vi "Display Info.vi"(7 "Layout ref":refnum<vi>, 8 "error in (no error)":errorcluster, 9 "Modify (F) /Add [T]":bool, 10 "Names in use":string[](array[string]), 11 "ArduinoDAC in":refnum<class "ArduinoDAC.lvclass">) -> (0 "error out":errorcluster, 1 "Names in use out":string[](array[string]), 2 "Changes Made?":bool, 3 "ArduinoDAC out":refnum<class "ArduinoDAC.lvclass">)   [LabVIEW 2013, in "ArduinoDAC.lvclass"]
uses:
  ArduinoDAC.lvclass
  TypeDefs/ColumnAppearCluster.ctl
  ArduinoDAC.lvclass/ArduinoDAC.ctl
  ColumnVIs/Column/Column.lvclass
panel:
  in  "Steps Column Appearance":T1={"Column Name"="Frequency", "Width"=30, "Bkgd"=[16448250], "Text"=[0]}
  in  "EndV Column Appearance":T1={"Column Name"="Frequency", "Width"=30, "Bkgd"=[16448250], "Text"=[0]}
  in  "StartV Column Appearance":T1={"Column Name"="Frequency", "Width"=30, "Bkgd"=[16448250], "Text"=[0]}
  in  "Device Description":string
  in  "Hardware Settings":T2={"PB Trigger Line"=65535, "Serial Port"=""}
  in  "Name":string
  in  "Done":bool
  in  "Cancel":bool
  # "This VI just sets the wiring structure.\nOpen a child override version instead!"
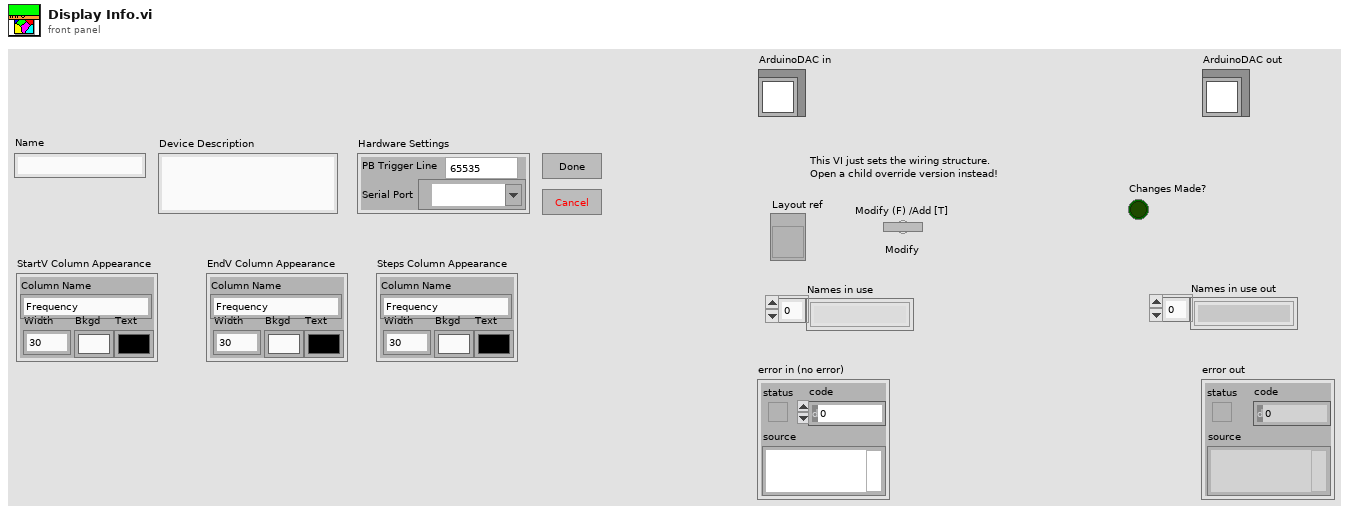
[diagram p1: front panel]
types:
  T1 = typedef "ColumnAppearCluster.ctl" = cluster{"Column Name":string, "Width":u32, "Bkgd":u32[], "Text":u32[]}
  T2 = cluster{"PB Trigger Line":u16, "Serial Port":refnum<visa-resource-name>}
  T3 = cluster{u16, "Serial Port":refnum<visa-resource-name>}
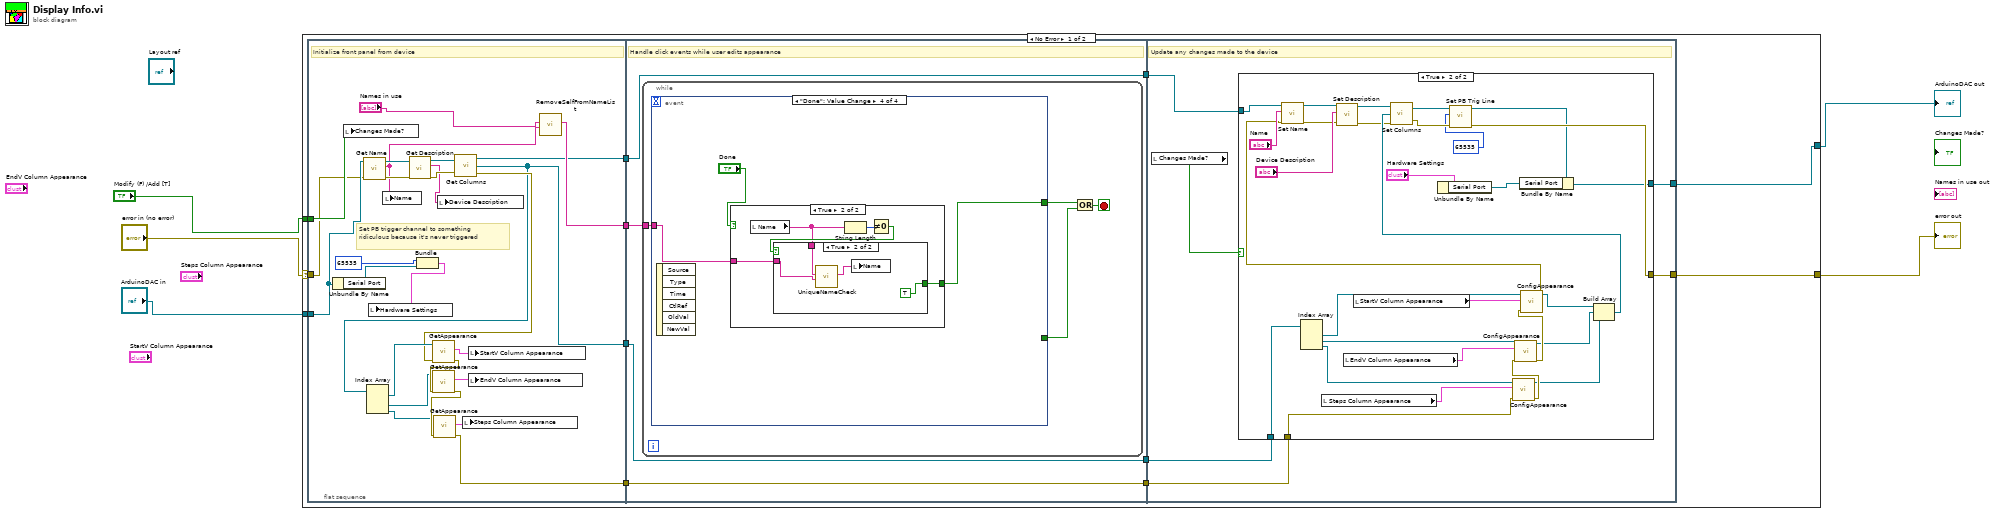
[diagram p0: block diagram]
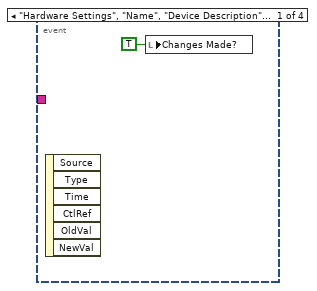
[diagram p2: hidden frame]
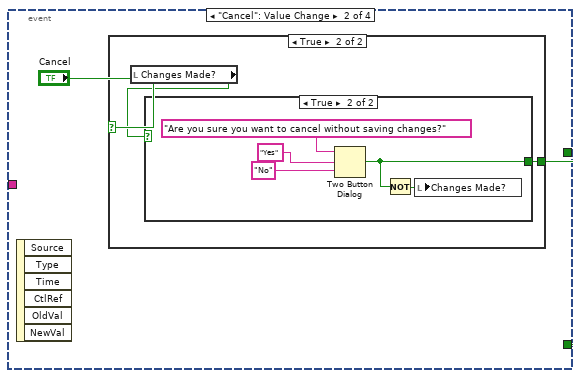
[diagram p3: hidden frame]
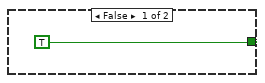
[diagram p5: hidden frame]
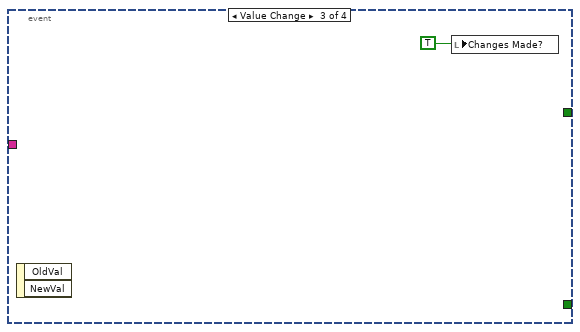
[diagram p6: hidden frame]
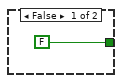
[diagram p7: hidden frame]
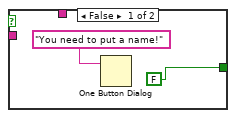
[diagram p8: hidden frame]
diagram:
  n1 = case shown="No Error" "error in (no error)" {
    selector: "error in (no error)" -> [w15 w119]
    tunnel: [w7 w119] -> w1
    tunnel: [w6 w118] -> w2
    tunnel: "ArduinoDAC in" -> [w16 w118]
    tunnel: "Modify (F) /Add [T]" -> [w17 _]
    frame No Error {
      n2 = flat-sequence {
        tunnel: w17 -> [w43]
        tunnel: w16 -> [w39]
        tunnel: w15 -> [w37]
        tunnel: [w28] -> w14
        tunnel: [w27] -> w13
        tunnel: [w26] -> w11
        tunnel: [w20] -> w9
        tunnel: w14 -> [w47]
        tunnel: w13 -> [w46]
        tunnel: [w46] -> w12
        tunnel: w11 -> [w45]
        tunnel: [w45] -> w10
        tunnel: w9 -> [w44]
        tunnel: [w44] -> w8
        tunnel: w12 -> [w85]
        tunnel: w10 -> [w84]
        tunnel: w8 -> [w83]
        tunnel: [w81] -> w7
        tunnel: [w80] -> w6
        frame #0 {
          # "Set PB trigger channel to something ridiculous because it's never triggered"
          # "Initialize front panel from device"
          n3 = Unbundle By Name(w39) -> ("Serial Port"=w41:refnum<visa-resource-name>)
          n4 = local write "Changes Made?"(w43) -> ()
          n5 = call-dynamic "Get Name.vi"("error in (no error)"=w37, "Device in"=w39) -> ("error out"=w36:errorcluster, "Name"=w33:string, "Device out"=w38:refnum<class "ArduinoDAC.lvclass">)  [unwired: 7 in]
          n6 = local write "Name"(w33) -> ()
          n7 = call-dynamic "Get Description.vi"("error in (no error)"=w36, "Device in"=w38) -> ("error out"=w34:errorcluster, "Device Description"=w32:string, "Device out"=w35:refnum<class "ArduinoDAC.lvclass">)  [unwired: 7 in]
          n8 = Bundle(u16 65535, "Serial Port"=w41) -> (w40:T3)  [unwired: 1 in]
          n9 = local write "Hardware Settings"(w40) -> ()
          n10 = local write "Device Description"(w32) -> ()
          n11 = call-dynamic "Get Columns.vi"("Device in"=w35, "error in (no error)"=w34) -> ("Device out"=w27:refnum<class "ArduinoDAC.lvclass">, "Columns"=w26:refnum<class "Column.lvclass">[], "error out"=w30:errorcluster)
          n12 = Index Array(array=w26) -> (element #1=w31:refnum<class "Column.lvclass">, element #2=w23:refnum<class "Column.lvclass">, element #3=w21:refnum<class "Column.lvclass">)  [unwired: 3 in]
          n13 = call "GetAppearance.vi"("error in (no error)"=w30, "Column in"=w31) -> ("error out"=w24:errorcluster, "Column Appearance"=w29:T1)  [unwired: 7 in, 1 out]
          n14 = call "GetAppearance.vi"("error in (no error)"=w24, "Column in"=w23) -> ("error out"=w22:errorcluster, "Column Appearance"=w19:T1)  [unwired: 7 in, 1 out]
          n15 = call "GetAppearance.vi"("error in (no error)"=w22, "Column in"=w21) -> ("error out"=w20:errorcluster, "Column Appearance"=w18:T1)  [unwired: 7 in, 1 out]
          n16 = local write "Steps Column Appearance"(w18) -> ()
          n17 = local write "StartV Column Appearance"(w29) -> ()
          n18 = local write "EndV Column Appearance"(w19) -> ()
          n19 = call "RemoveSelfFromNameList.vi"("self Name"=w33, "Names in use"="Names in use") -> ("Reserved Names"=w28:string[])  [unwired: 9 in]
        }
        frame #1 {
          # "Handle click events while user edits appearance"
          n20 = while {
            tunnel: w47 -> [w48]
            stop <- w51 stop-if-true
            n21 = event shown="[3] \"Done\": Value Change" {
              selector: _ -> [_ _ _ _]
              dyn-events: _ -> [_ _ _ _]
              timeout: _ -> [_ _ _ _]
              tunnel: [_ w54 _ _] -> w50
              tunnel: [_ _ _ w67] -> w49
              tunnel: w48 -> [_ _ _ w65]
              event "Hardware Settings", "Name", "Device Description": Value Change {
                n22 = event-data() -> ()  [unwired: 1 in, 6 out]
                n23 = local write "Changes Made?"(TRUE ("Changes Made?")) -> ()
              }
              event "Cancel": Value Change {
                n24 = event-data() -> ()  [unwired: 1 in, 6 out]
                n25 = case shown="True" "Cancel" {
                  selector: "Cancel" -> [w55 _]
                  tunnel: [w55 w57] -> w54
                  frame False {
                  }
                  frame True {
                    n26 = local read "Changes Made?"() -> (w56:bool)
                    n27 = case shown="True" w56 {
                      tunnel: [TRUE w60] -> w57
                      frame False {
                      }
                      frame True {
                        n28 = Two Button Dialog(message="Are you sure you want to cancel without saving changes?", 1:"No", 2:"Yes") -> (T button?=w60:bool)
                        n29 = Not(x=w60) -> (.not. x?=w59:bool)
                        n30 = local write "Changes Made?"(w59) -> ()
                      }
                    }
                  }
                }
              }
              event Value Change {
                n31 = event-data() -> ()  [unwired: 1 in, 2 out]
                n32 = local write "Changes Made?"(TRUE) -> ()
              }
              event "Done": Value Change {
                n33 = event-data() -> ()  [unwired: 1 in, 6 out]
                n34 = case shown="True" "Done" {
                  tunnel: [FALSE w71] -> w67
                  tunnel: w65 -> [_ w70]
                  frame False {
                  }
                  frame True {
                    n35 = local read "Name"() -> (w69:string)
                    n36 = String Length(string=w69) -> (length=w73:i32)
                    n37 = Not Equal To 0?(x=w73) -> (x != 0?=w72:bool)
                    n38 = case shown="True" w72 {
                      tunnel: [FALSE TRUE] -> w71
                      tunnel: w70 -> [_ w78]
                      tunnel: w69 -> [_ w77]
                      frame False {
                        n39 = One Button Dialog(message="You need to put a name!") -> ()  [unwired: 1 in, 1 out]
                      }
                      frame True {
                        n40 = call "UniqueNameCheck.vi"("Names in use"=w78, "Device Name"=w77) -> ("Unique name"=w76:string)  [unwired: 8 in, 1 out]
                        n41 = local write "Name"(w76) -> ()
                      }
                    }
                  }
                }
              }
            }
            n42 = Or(x=w49, y=w50) -> (x .or. y?=w51:bool)
          }
        }
        frame #2 {
          # "Update any changes made to the device"
          n43 = local read "Changes Made?"() -> (w82:bool)
          n44 = case shown="True" w82 {
            tunnel: w85 -> [w87 w117]
            tunnel: w84 -> [_ w112]
            tunnel: w83 -> [w86 w96]
            tunnel: [w86 w101] -> w81
            tunnel: [w87 w98] -> w80
            frame False {
            }
            frame True {
              n45 = Index Array(array=w112) -> (element #1=w111:refnum<class "Column.lvclass">, element #2=w93:refnum<class "Column.lvclass">, element #3=w92:refnum<class "Column.lvclass">)  [unwired: 3 in]
              n46 = local read "Steps Column Appearance"() -> (w90:T1)
              n47 = local read "EndV Column Appearance"() -> (w91:T1)
              n48 = local read "StartV Column Appearance"() -> (w108:T1)
              n49 = Unbundle By Name("Hardware Settings") -> ("Serial Port"=w99:refnum<visa-resource-name>)
              n50 = call "ConfigAppearance.vi"("error in (no error)"=w96, "Column Appearance"=w90, "Column in"=w92) -> ("error out"=w95:errorcluster, "Column out"=w88:refnum<class "Column.lvclass">)  [unwired: 7 in]
              n51 = call "ConfigAppearance.vi"("error in (no error)"=w95, "Column Appearance"=w91, "Column in"=w93) -> ("error out"=w94:errorcluster, "Column out"=w89:refnum<class "Column.lvclass">)  [unwired: 7 in]
              n52 = call "ConfigAppearance.vi"("error in (no error)"=w94, "Column Appearance"=w108, "Column in"=w111) -> ("error out"=w110:errorcluster, "Column out"=w107:refnum<class "Column.lvclass">)  [unwired: 7 in]
              n53 = call-dynamic "Set Name.vi"("error in (no error)"=w110, "Name"="Name", "Device in"=w117) -> ("error out"=w109:errorcluster, "Device out"=w115:refnum<class "ArduinoDAC.lvclass">)  [unwired: 7 in]
              n54 = call-dynamic "Set Description.vi"("error in (no error)"=w109, "Device Description"="Device Description", "Device in"=w115) -> ("error out"=w104:errorcluster, "Device out"=w105:refnum<class "ArduinoDAC.lvclass">)  [unwired: 7 in]
              n55 = Build Array(w107, w89, w88) -> (w106:refnum<class "Column.lvclass">[])
              n56 = call-dynamic "Set Columns.vi"("error in (no error)"=w104, "Columns"=w106, "Device in"=w105) -> ("error out"=w102:errorcluster, "Device out"=w103:refnum<class "ArduinoDAC.lvclass">)  [unwired: 1 in]
              n57 = call-dynamic "Set PB Trig Line.vi"("error in (no error)"=w102, "PB Trigger Line"=u16 65535, "Device in"=w103) -> ("error out"=w101:errorcluster, "Device out"=w100:refnum<class "ArduinoDAC.lvclass">)  [unwired: 7 in]
              n58 = Bundle By Name(cluster=w100, "Serial Port"=w99) -> (w98:refnum<class "ArduinoDAC.lvclass">)
            }
          }
        }
      }
    }
    frame Error {
    }
  }
  "error out" <- w1
  "ArduinoDAC out" <- w2
